vi "Single Float Multi Test.vi"() -> ()   [LabVIEW 2021]
uses:
  Source/Omni-Bus/Omni_Bus.lvclass
  Source/Omni-Bus/Support/Broad Types.ctl
  Source/Local Bus/Local Bus.lvclass
  C:/TSA/Omni-Bus/Source/Omni-Bus/Bus Access/Bus_Access.lvclass
  <vilib>/Utility/Data Type/Type Definitions/Data Type.ctl
  <vilib>/TSA/Abstract Data Classes/Abs_Types/Type/Abs_Type.lvclass/Abs_Type.ctl
  Source/Omni-Bus/Omni_Bus.lvclass/Omni_Bus.ctl
  Source/Omni-Bus/Support/Write/Write Multi SGL.vi
  Source/Omni-Bus/Support/Read As/Read Multi Numeric as U64.vi
  Source/Omni-Bus/Support/Get/Get Multi SGL.vi
  Source/Omni-Bus/Support/FindMultiVar.vi
  Source/Omni-Bus/Support/FindVar.vi
  <vilib>/Utility/error.llb/Clear Errors.vi
  <vilib>/TSA/Abstract Data Classes/Abs_Types/Type/Properties/Write Tag.vi
  Source/Omni-Bus/Properties/Read Var Map.vi
  <vilib>/TSA/Abstract Data Classes/Abs_Types/Type/Properties/Read Tag.vi
  <vilib>/TSA/Abstract Data Classes/Abs_Types/Single Float/Abs_Single Float.lvclass
  C:/Program Files (x86)/National Instruments/LabVIEW 2021/vi.lib/TSA/Abstract Data Classes/Abs_Types/Type/Abs_Type.lvclass
  <vilib>/TSA/Abstract Data Classes/Abs_Types/Value/Abs_Value.lvclass
  Source/Omni-Bus/Support/Check For Read Only Error.vi
  Source/Omni-Bus/Support/Incorrect Tag String Error.vi
  <vilib>/TSA/Abstract Data Classes/Abs_Types/Type/Abs_Type.lvclass
  <vilib>/TSA/Abstract Data Classes/Abs_Types/Numeric/Abs_Numeric.lvclass
  <vilib>/Utility/Data Type/NI_Data Type.lvlib
  Source/Omni-Bus/Support/Read/Read Multi SGL.vi
panel:
  out "Singles":u64[](array[numeric])
  in  "Array":sgl[](array[numeric])
  out "error out 3":errorcluster
  out "error out 2":errorcluster
  in  "Tag 2":string[](array[combo])
  in  "stop":bool
  in  "Tags":string[](array[combo])
  out "error out":errorcluster
  out "Tags":string[](array[string])
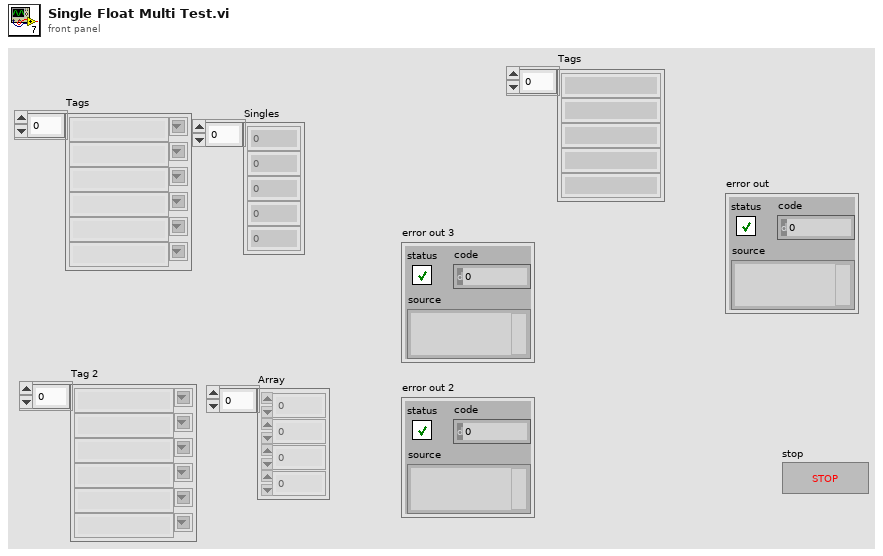
[diagram p1: front panel]
types:
  T1 = typedef "NI_Data Type.lvlib/Data Type.ctl" = enum8{"Invalid Type", "Void", "I8", "I16", "I32", "I64", "U8", "U16", "U32", "U64", "Single Float", "Double Float", "Extended Float", "Single Complex", "Double Complex", "Extended Complex", "Enum U8", "Enum U16", "Enum U32", "Enum U64", "Single Float With Unit", "Double Float With Unit", "Extended Float With Unit", "Single Complex with Unit", "Double Complex with Unit", "Extended Complex with Unit", "Boolean", "String", "Path", "Picture", "Tag", "Array", "Cluster", "Variant", "LV Variant", "Waveform", "Timestamp", "Digital Waveform", "Digital Data", "ExpressData", "Refnum", "External Data", "VI", "Poly VI", "LabVIEW Class Instance", "Fixed Point", "Set Collection", "Map Collection"}
  T2 = typedef "Omni_Bus.lvclass/Broad Types.ctl" = enum16{"All Tags", "NI Specific Type", "Boolean", "String", "Numeric", "Float", "Integer", "Collection", "All Value Types", "Non Value Types"}
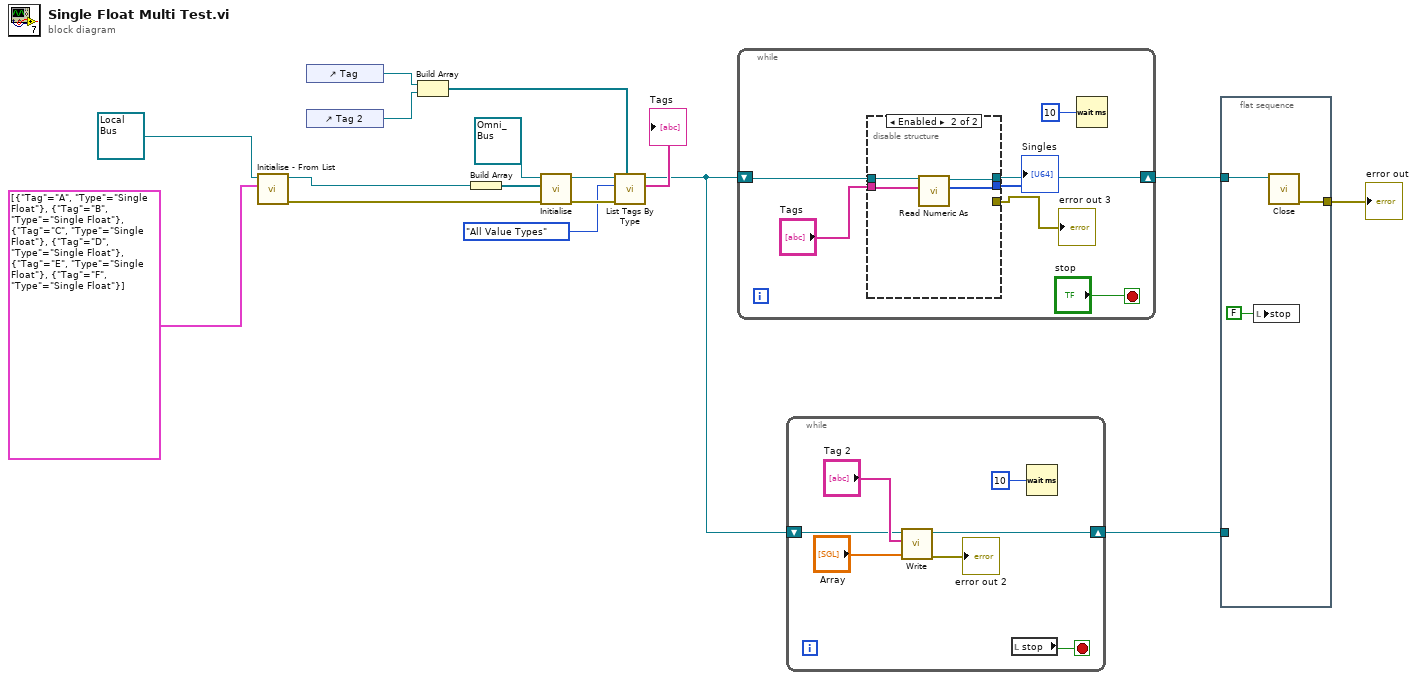
[diagram p0: block diagram]
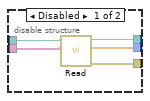
[diagram p2: hidden frame]
diagram:
  n1 = call "Initialise - From List.vi"("Tag List"=cluster{"Tag":string, "Type":T1}[] [{"Tag"="A", "Type"=enum."Single Float"}, {"Tag"="B", "Type"=enum."Single Float"}, {"Tag"="C", "Type"=enum."Single Float"}, {"Tag"="D", "Type"=enum."Single Float"}, {"Tag"="E", "Type"=enum."Single Float"}, {"Tag"="F", "Type"=enum."Single Float"}], "Local Bus in"=refnum<class "Local Bus.lvclass"> refnum ("Local Bus.lvclass")) -> ("error out"=w6:errorcluster, "Local Bus out"=w7:refnum<class "Local Bus.lvclass">)  [unwired: 8 in]
  n2 = control-ref of="Tag"() -> (w3:refnum<vi>)
  n3 = control-ref of="Tag 2"() -> (w2:refnum<vi>)
  n4 = Build Array(w3, w2) -> (w1:refnum<vi>[])
  n5 = Build Array(w7) -> (w16:refnum<class "Local Bus.lvclass">[])
  n6 = call-dynamic "Initialise.vi"("error in (no error)"=w6, "Bus Access"=w16, "Var Bus in"=refnum<class "Omni_Bus.lvclass"> refnum) -> ("error out"=w14:errorcluster, "Var Bus out"=w15:refnum<class "Omni_Bus.lvclass">)  [unwired: 7 in]
  n7 = call "List Tags By Type.vi"("Combo Boxes"=w1, "error in (no error)"=w14, "Broad Types"=Broad_Types."All Value Types", "Var Bus in"=w15) -> ("Tags"=→"Tags":string[], "Var Bus out"=w9:refnum<class "Omni_Bus.lvclass">)  [unwired: 4 in, 2 out]
  n8 = while {
    shift-right: [w21] -> w10
    shift-left: w9 -> [w22]
    stop <- "stop" stop-if-true
    n9 = disable-structure shown="Enabled" {
      disable-tunnel: w22 -> [w29 w33]
      disable-tunnel: [w28 w32] -> w21
      disable-tunnel: "Tags" -> [w27 w30]
      disable-tunnel: [w26 _] -> w19
      disable-tunnel: [w25 w31] -> w18
      frame Disabled {
        n10 = call-poly "Read.vi"("Tag"=w27, "Var Bus in"=w29) -> ("error out"=w26:errorcluster, "Singles"=w25:sgl[], "Var Bus out"=w28:refnum<class "Omni_Bus.lvclass">)  [unwired: 7 in]
      }
      frame Enabled {
        n11 = call-poly "Read Numeric As.vi"("Tag"=w30, "Var Bus in"=w33) -> ("Array"=w31:u64[], "Var Bus out"=w32:refnum<class "Omni_Bus.lvclass">)  [unwired: 7 in, 1 out]
      }
    }
    "error out 3" <- w19
    "Singles" <- w18
    n12 = Wait (ms)(milliseconds to wait=u32 10) -> ()  [unwired: 1 out]
  }
  n13 = while {
    shift-right: [w36] -> w8
    shift-left: w9 -> [w37]
    stop <- w40 stop-if-true
    n14 = call-poly "Write.vi"("Array"="Array", "Tag"="Tag 2", "Omni_Bus in"=w37) -> ("error out"=→"error out 2":errorcluster, "Omni_Bus out"=w36:refnum<class "Omni_Bus.lvclass">)  [unwired: 7 in]
    n15 = local read "stop"() -> (w40:bool)
    n16 = Wait (ms)(milliseconds to wait=u32 10) -> ()  [unwired: 1 out]
  }
  n17 = flat-sequence {
    tunnel: [w43] -> w11
    tunnel: w10 -> [w42]
    tunnel: w8 -> [_]
    frame #0 {
      n18 = local write "stop"(FALSE ("stop")) -> ()
      n19 = call-dynamic "Close.vi"("Data in"=w42) -> ("error out"=w43:errorcluster)  [unwired: 9 in, 1 out]
    }
  }
  "error out" <- w11
